vi "Set Channel Value (Red).vi"(8 "error in (no error)":errorcluster, 10 "Value":u8, 11 "ARGB Image":T1) -> (0 "error out":errorcluster, 3 "ARGB Image (Duplicate)":T1)   [LabVIEW 2020, in "image.lvlib"]
uses:
  image.lvlib
  ARGB Image.ctl
  ARGBChannels.ctl
  common/Module Path.vi
  <vilib>/Utility/error.llb/Error Cluster From Error Code.vi
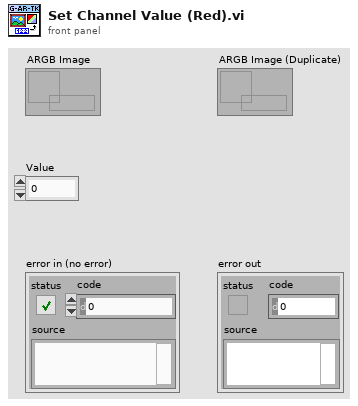
[diagram p1: front panel]
types:
  T1 = typedef "image.lvlib/ARGB Image.ctl" = refnum<data-value>
  T2 = typedef "image.lvlib/ARGBChannels.ctl" = enum8{"Blue", "Green", "Red", "Alpha"}
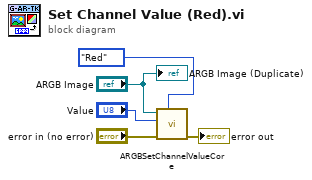
[diagram p0: block diagram]
diagram:
  n1 = call "ARGBSetChannelValueCore.vi"("Channel"=ARGBChannels."Red" ("Extract_Operation"), "error in (no error)"="error in (no error)", "Value"="Value", "Src"="ARGB Image") -> ("error out"=→"error out":errorcluster)  [unwired: 7 in]
  "ARGB Image (Duplicate)" <- "ARGB Image"
